vi "Debug - Verbose - File Path--FGV.vi"() -> (3 "Debug Pathname":path)   [LabVIEW 2017, in "Communications Library.lvlib"]
doc: "The pathname of the debug file is generated and stored in a functional global variable.\n\nOn the first run of this vi;\n-A unique filename is generated\n-The creation time of the file is logged\n-The file is closed\n\nOn subsequent runs of this vi;\n-The previously used pathname is returned\n\nNote: This VI must always be run in non reenterant mode."
uses:
  Communications Library.lvlib
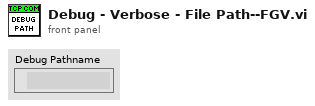
[diagram p1: front panel]
types:
  T1 = enum16{"open", "replace", "create", "open or create", "replace or create", "replace or create with confirmation"}
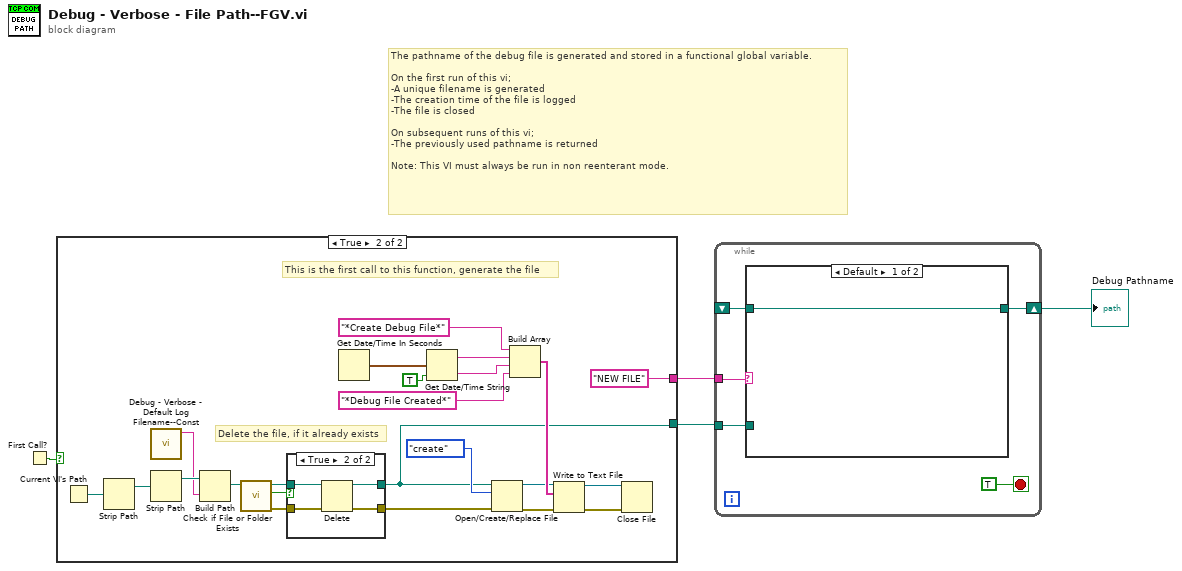
[diagram p0: block diagram]
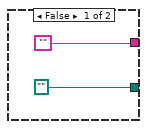
[diagram p2: hidden frame]
diagram:
  # "The pathname of the debug file is generated and stored in a functional global variable.\n\nOn the first run of this vi;\n-A unique filename is generated\n-The creation time of the file is logged\n-The file is closed\n\nOn subsequent runs of this vi;\n-The previously used pathname is returned\n\nNote: This VI must always be run in non reenterant mode."
  n1 = First Call?() -> (First Call?: T/F=w4:bool)
  n2 = case shown="True" w4 {
    tunnel: [path "" w9] -> w2
    tunnel: ["" "NEW FILE"] -> w3
    frame False {
    }
    frame True {
      # "Delete the file, if it already exists"
      # "This is the first call to this function, generate the file"
      n3 = Current VI's Path() -> (path=w28:path)
      n4 = Strip Path(path=w28) -> (stripped path=w29:path)  [unwired: 1 out]
      n5 = call "Debug - Verbose - Default Log Filename--Const.vi"() -> ("Debug Log Filename"=w16:string)  [unwired: 11 in]
      n6 = Strip Path(path=w29) -> (stripped path=w17:path)  [unwired: 1 out]
      n7 = Build Path(base path=w17, name or relative path=w16) -> (appended path=w10:path)
      n8 = call <vilib>:"Check if File or Folder Exists.vi"("path"=w10) -> ("error out"=w13:errorcluster, "file or folder exists?"=w15:bool, "dup path"=w12:path)  [unwired: 8 in]
      n9 = case shown="True" w15 {
        tunnel: [w31 w35] -> w9
        tunnel: w12 -> [w31 w34]
        tunnel: w13 -> [w30 w33]
        tunnel: [w30 w32] -> w14
        frame False {
        }
        frame True {
          n10 = Delete(path (use dialog)=w34, error in=w33) -> (deleted path=w35:path, error out=w32:errorcluster)  [unwired: 3 in, 1 out]
        }
      }
      n11 = Get Date/Time In Seconds() -> (seconds since 1Jan1904=w21:timestamp)
      n12 = Get Date/Time String(seconds (now)=w21, want seconds? (F)=TRUE) -> (date string=w20:string, time string=w19:string)  [unwired: 1 in]
      n13 = Open/Create/Replace File(file path (use dialog)=w9, error in=w14, operation (0:open)=T1."create") -> (refnum out=w8:refnum<file>, error out=w7:errorcluster)  [unwired: 3 in, 1 out]
      n14 = Build Array("*Create Debug File*", w20, w19, "*Debug File Created*") -> (w25:string[])
      n15 = Write to Text File(file (use dialog)=w8, text=w25, error in=w7) -> (refnum out=w23:refnum<file>, error out=w24:errorcluster)  [unwired: 1 in, 1 out]
      n16 = Close File(refnum=w23, error in=w24) -> ()  [unwired: 2 out]
    }
  }
  n17 = while {
    tunnel: w3 -> [w40]
    tunnel: w2 -> [w39]
    shift-right: [w38] -> w1
    shift-left: _ -> [w37]
    stop <- TRUE stop-if-true
    n18 = case shown="Default" w40 {
      tunnel: w39 -> [_ w42]
      tunnel: [w41 w42] -> w38
      tunnel: w37 -> [w41 _]
      frame Default {
      }
      frame "NEW FILE" {
      }
    }
  }
  "Debug Pathname" <- w1
